vi "initialize_instruments_discharge (SubVI).vi"(0 "Sample rate":dbl=1000.0 format="%0.2f", 5 "Electrode outupt channels":tag="Dev4/ao0") -> (4 "SampClk.Rate":dbl, 6 "electrode_config":T1)   [LabVIEW 2018]
uses:
  <vilib>/DAQmx/create/channels.llb/DAQmx Create Channel (AO-Voltage-Basic).vi
  <vilib>/DAQmx/configure/timing.llb/DAQmx Timing (Sample Clock).vi
  <resource>/objmgr/daqmx.rc
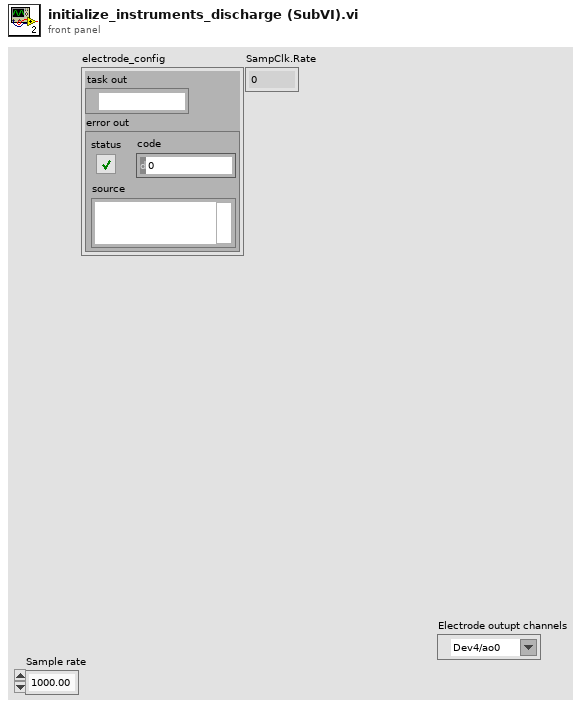
[diagram p1: front panel]
types:
  T1 = cluster{"task out":refnum<k21>, "error out":errorcluster}
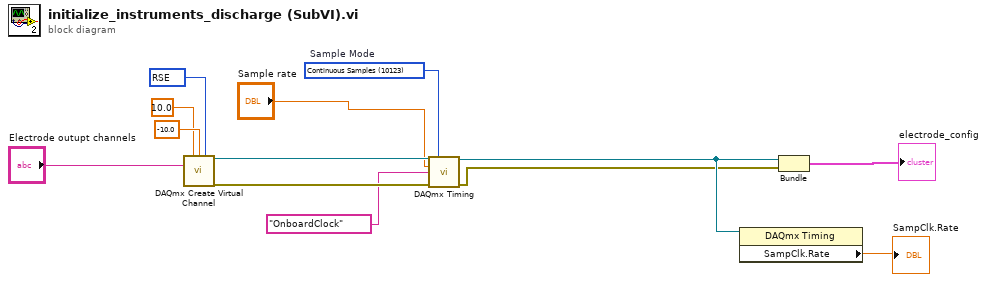
[diagram p0: block diagram]
diagram:
  w8 = 10083 items=["Default"=-1, "RSE"=10083, "Differential"=10106, "Pseudodifferential"=12529] ("output terminal configuration")
  w13 = 10123 items=["Finite Samples"=10178, "Continuous Samples"=10123, "Hardware Timed Single Point"=12522]  # Sample Mode
  n1 = call-poly <vilib>:"DAQmx Create Virtual Channel.vi"("maximum value"=10.0, "minimum value"=-10.0, "output terminal configuration"=w8, "physical channels"="Electrode outupt channels") -> ("task out"=w11:refnum<k21>, "error out"=w12:errorcluster)  [unwired: 10 in]
  n2 = call-poly <vilib>:"DAQmx Timing.vi"("task/channels in"=w11, "sample mode"=w13, "rate"="Sample rate", "source"=tag "OnboardClock" ("Sample Clock Source"), "error in"=w12) -> ("task out"=w4:refnum<k21>, "error out"=w3:errorcluster)  [unwired: 9 in]
  n3 = property class="DAQmx Timing"(reference=w4) -> ("SampClk.Rate"=→"SampClk.Rate":dbl)  [unwired: 1 in, 2 out]
  n4 = Bundle("task out"=w4, "error out"=w3) -> (→"electrode_config":T1)  [unwired: 1 in]
